vi "Get Result.vi"(6 "Last request":bool, 8 "error in (no error)":errorcluster, 11 "Process Object in":refnum<class "Process Object.lvclass">) -> (0 "error out":errorcluster, 2 "Result":refnum<class "Acquired Result.lvclass">, 3 "Process Object out":refnum<class "Process Object.lvclass">)   [LabVIEW 2016, in "Process Object.lvclass"]
uses:
  Process Object.lvclass
  NHMFL_Core/Libraries/Instruments/Results/Acquired Result/Acquired Result.lvclass
  Process Object.lvclass/Process Object.ctl
  Read Result.vi
  Read Result ready.vi
  Write Result ready.vi
  Worker/Worker.lvclass
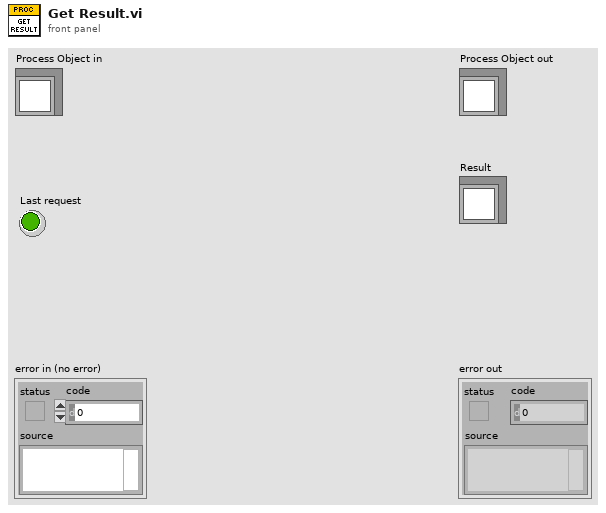
[diagram p1: front panel]
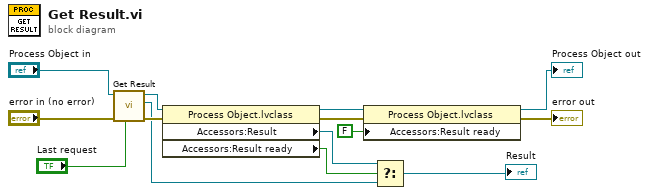
[diagram p0: block diagram]
diagram:
  n1 = call-parent "Get Result.vi"("Last request"="Last request", "error in (no error)"="error in (no error)", "Worker in"="Process Object in") -> ("error out"=w14:errorcluster, "Result"=w5:refnum<class "Acquired Result.lvclass">, "Worker out"=w9:refnum<class "Process Object.lvclass">)  [unwired: 6 in]
  n2 = property class="Process Object.lvclass"(reference=w9, error in=w14) -> (reference out=w3:refnum<class "Process Object.lvclass">, error out=w10:errorcluster, "Accessors:Result"=w8:refnum<class "Acquired Result.lvclass">, "Accessors:Result ready"=w7:bool)
  n3 = property class="Process Object.lvclass"(reference=w3, error in=w10, "Accessors:Result ready"=FALSE ("Result ready")) -> (reference out=→"Process Object out":refnum<class "Process Object.lvclass">, error out=→"error out":errorcluster)
  n4 = Select(t=w8, s=w7, f=w5) -> (s? t:f=→"Result":refnum<class "Acquired Result.lvclass">)
